vi "RunPython.vi"(7 "keep cmd window open (f)":bool, 10 "PathToScript":path) -> (0 "error out":errorcluster, 2 "standard output":string)   [LabVIEW 2017, in "LV-PY.lvlib"]
uses:
  LV-PY.lvlib
  Framework/Config_class/Config.lvclass/Config.ctl
  Framework/Config_class/Accessors/Read PARTF Root Directory.vi
  Framework/Config_class/Config.lvclass
panel:
  out "concatenated string":string
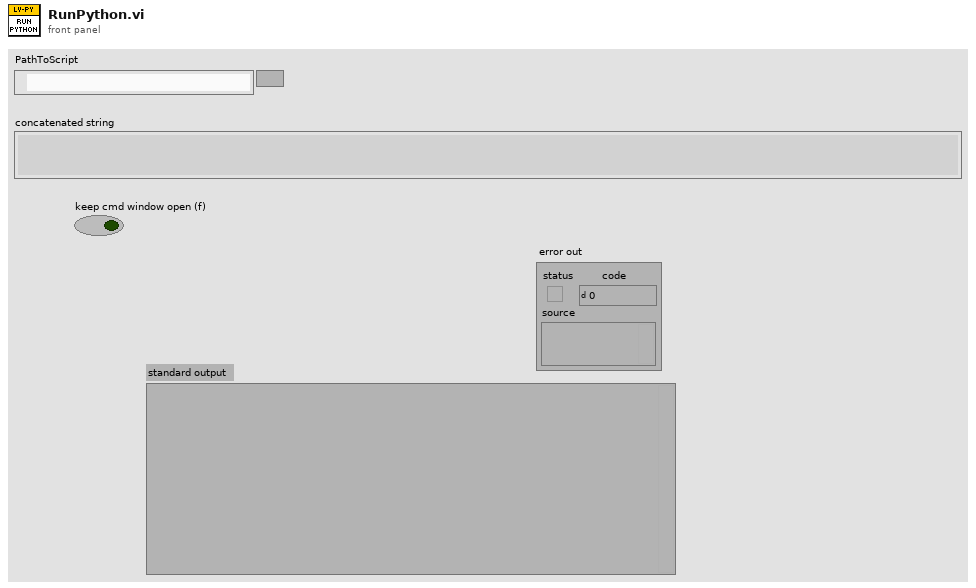
[diagram p1: front panel]
types:
  T1 = typedef "Framework.lvlib/Config.lvclass/RootDir.ctl" = cluster{"pathRootDir":path, "btnOutPath":bool, "OutDir":string, "btnOpenOutputDir":bool, "ScriptDir":string, "btnOpenScriptDir":bool, "TestDir":string, "btnOpenTestDir":bool}
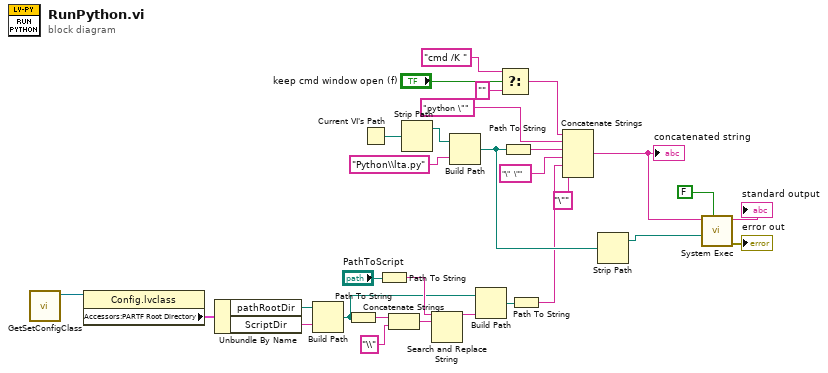
[diagram p0: block diagram]
diagram:
  n1 = call "GetSetConfigClass.vi"() -> ("Ref out"=w12:refnum<class "Config.lvclass">)  [unwired: 11 in]
  n2 = property class="Config.lvclass"(reference=w12) -> ("Accessors:PARTF Root Directory"=w11:T1)  [unwired: 1 in, 2 out]
  n3 = Unbundle By Name(w11) -> ("pathRootDir"=w4:path, "ScriptDir"=w10:string)
  n4 = Build Path(base path=w4, name or relative path=w10) -> (appended path=w1:path)
  n5 = Path To String(path=w1) -> (string=w8:string)
  n6 = Current VI's Path() -> (path=w30:path)
  n7 = Path To String(path="PathToScript") -> (string=w6:string)
  n8 = Concatenate Strings(w8, "\\" ("string")) -> (w7:string)
  n9 = Strip Path(path=w30) -> (stripped path=w24:path)  [unwired: 1 out]
  n10 = Search and Replace String(input string=w6, search string=w7) -> (result string=w5:string)  [unwired: 6 in, 3 out]
  n11 = Build Path(base path=w24, name or relative path="Python\\lta.py") -> (appended path=w22:path)
  n12 = Build Path(base path=w1, name or relative path=w5) -> (appended path=w3:path)
  n13 = Select(t="cmd /K " ("string"), s="keep cmd window open (f)", f="") -> (s? t:f=w15:string)
  n14 = Path To String(path=w22) -> (string=w28:string)
  n15 = Path To String(path=w3) -> (string=w2:string)
  n16 = Concatenate Strings(w15, "python \"" ("command line"), w28, "\"  \"" ("string"), w2, "\"" ("string")) -> (w23:string)
  "concatenated string" <- w23
  n17 = Strip Path(path=w22) -> (stripped path=w21:path)  [unwired: 1 out]
  n18 = call <vilib>:"System Exec.vi"("wait until completion? (T)"=FALSE, "working directory"=w21, "command line"=w23) -> ("error out"=→"error out":errorcluster, "standard output"=→"standard output":string)  [unwired: 5 in, 2 out]
